vi "Response Error Checker.vi"(8 "error in (no error)":errorcluster, 10 "Response in":string, 11 "EPU452 in":refnum<class "EPU452.lvclass">) -> (0 "error out":errorcluster, 2 "Response out":string, 3 "EPU452 out":refnum<class "EPU452.lvclass">)   [LabVIEW 2018, in "EPU452.lvclass"]
uses:
  EPU452.lvclass
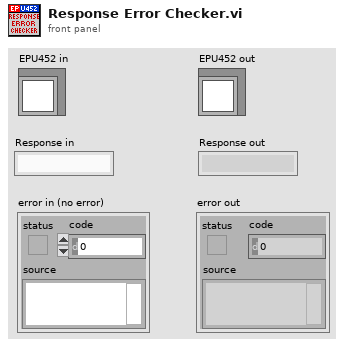
[diagram p1: front panel]
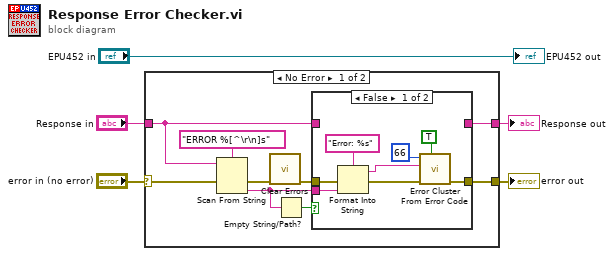
[diagram p0: block diagram]
diagram:
  n1 = case shown="No Error" "error in (no error)" {
    selector: "error in (no error)" -> [w8 w25]
    tunnel: [w9 w25] -> w4
    tunnel: "Response in" -> [w7 _]
    tunnel: [w6 _] -> w2
    frame No Error {
      n2 = Scan From String(format string="ERROR %[^\r\n]s", input string=w7, error in=w8) -> (error out=w11:errorcluster, output 1=w10:string)  [unwired: 2 in, 2 out]
      n3 = call <vilib>:"Clear Errors.vi"("error in (no error)"=w11) -> ("error out"=w12:errorcluster)  [unwired: 5 in, 1 out]
      n4 = Empty String/Path?(string/path=w10) -> (empty?=w13:bool)
      n5 = case shown="False" w13 {
        tunnel: w12 -> [w18 w24]
        tunnel: w10 -> [w17 _]
        tunnel: [w15 w24] -> w9
        tunnel: w7 -> [_ w23]
        tunnel: [_ w23] -> w6
        frame False {
          n6 = Format Into String(format string="Error: %s", error in=w18, w17) -> (resulting string=w16:string, error out=w19:errorcluster)  [unwired: 1 in]
          n7 = call <vilib>:"Error Cluster From Error Code.vi"("show call chain? (False)"=TRUE, "error in (no error)"=w19, "error message (\"\")"=w16, "error code (0)"=66) -> ("error out"=w15:errorcluster)  [unwired: 5 in]
        }
        frame True {
        }
      }
    }
    frame Error {
    }
  }
  "error out" <- w4
  "Response out" <- w2
  "EPU452 out" <- "EPU452 in"
